vi "Main.vi"() -> ()   [LabVIEW 2017]
uses:
  Acquisition/Hardware Configuration.ctl
  Settings/Settings.ctl
  Logging/Logging Configuration.ctl
  controls/UI Data.ctl
  controls/UI State.ctl
  <userlib>/Circular Buffer/Controls/Circular Buffer Operations.ctl
  <vilib>/Utility/miscctls.llb/LVStringsAndValuesArrayTypeDef.ctl
  <vilib>/measure/maresamp.llb/Resample N Waveforms (continuous).vi
  <userlib>/Circular Buffer/Instance VIs/Circular Buffer(2D Wfm-SGL with Attributes).vi
  <vilib>/Waveform/WDTOps.llb/WDT Number of Waveform Samples DBL.vi
  support/Message Queue/Enqueue Message (Single).vi
  <vilib>/Utility/error.llb/Error Cluster From Error Code.vi
  <vilib>/ErrorRing/Error Ring.xnode
  Acquisition/Acquisition.lvlib
  Logging/Logging.lvlib
  Settings/Settings.lvlib
  support/User Event - Stop/User Event - Stop.lvlib
  support/Message Queue/Message Queue.lvlib
  <userlib>/Circular Buffer/Circular Buffer.lvlib
  <vilib>/measure/NI_MAPro.lvlib
panel:
  out "Hardware Configuration":T1={"DAQmx Channel"="", "Sample Rate"=1000.0, "DAQmx Task"="", "ResetInterp"=FALSE, "GainConstants"=[2.0, 10.0, 1.0, 0.1, 0.01, 0.001], "FilterCoefficients"=[], "ChannelNames"=[], "ActiveChannels"=[], "Display Rate"=1000, "ResponseExtension"=TRUE}
  in  "Settings":bool
  in  "Start":bool
  in  "Trigger":bool caption="Force Trigger"
  out "Scale [mm/s]":u8(slide) max=0 scale=1.0..6.0
  out "Filter [Hz]":u8(slide) caption="Filter" max=0 scale=2.0..4.0
  in  "Autoscale":bool
  out "Status":string
  in  "Range Min":dbl=-10.0 format="%#_3f"
  in  "Range Max":dbl=10.0 format="%#_3f"
  in  "Chart Length[s]":dbl=10.0 min=1.0 max=120.0 step=1.0
  in  "Exit":bool
  out "WD":T2(array[cluster])
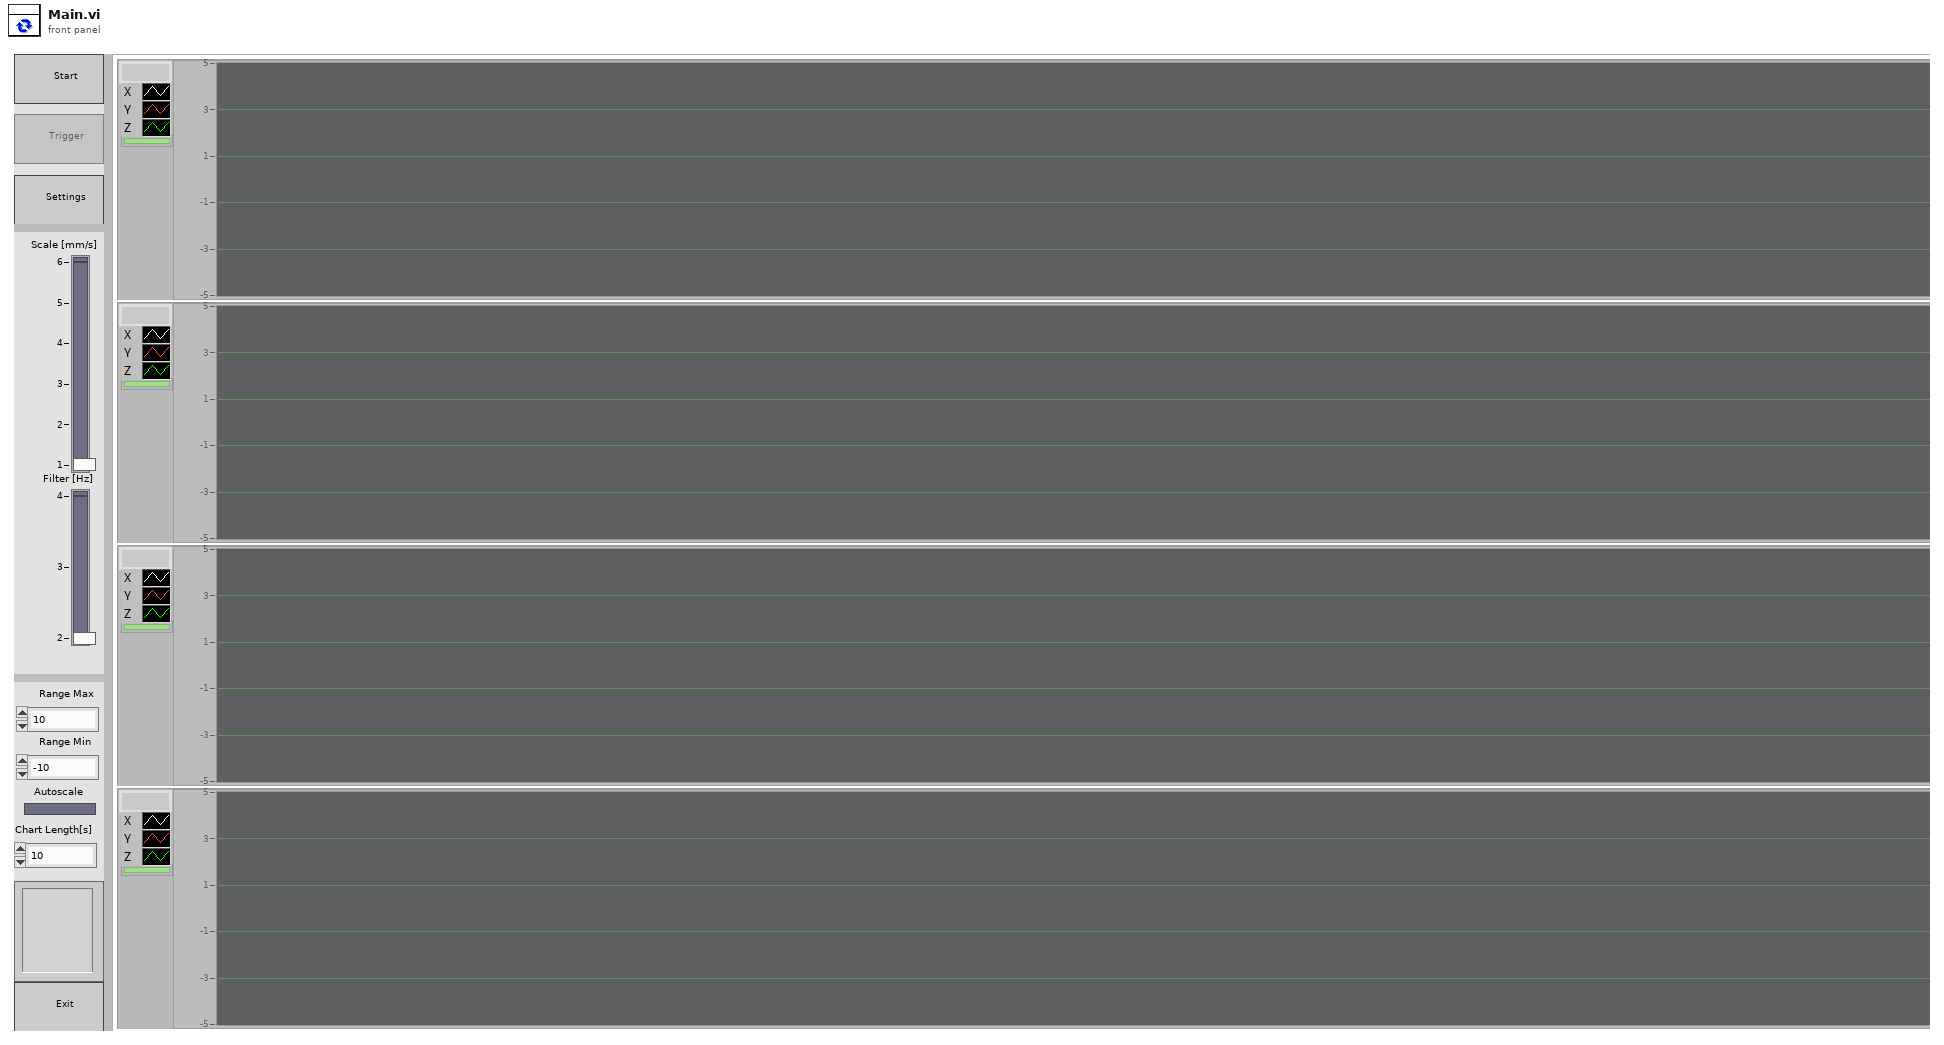
[diagram p1: front panel]
types:
  T1 = typedef "Acquisition.lvlib/Hardware Configuration.ctl" = cluster{"DAQmx Channel":string, "Sample Rate":dbl, "DAQmx Task":refnum<k21>, "ResetInterp":bool, "GainConstants":dbl[], "FilterCoefficients":dbl[][], "ChannelNames":string[], "ActiveChannels":i32[], "Display Rate":i32, "ResponseExtension":bool}
  T2 = cluster{"Graph":waveform(sgl)[], "Name 2":string, "Clip":bool}[]
  T3 = typedef "UI State.ctl" = enum16{"Idle", "Acquiring and Logging", "Waiting for Exit", "Waiting for Exit (Acq Stopped)", "Waiting for Exit (Log Stopped)", "Waiting for Stop", "Waiting for Stop (Acq Stopped)", "Waiting for Stop (Log Stopped)"}
  T4 = typedef "UI Data.ctl" = cluster{"Start Ref":refnum<vi>, "Trigger Ref":refnum<vi>, "Settings Ref":refnum<vi>, "Status Ref":refnum<vi>, "Exit Ref":refnum<vi>, "Data Ref":refnum<vi>}
  T5 = typedef "Settings.lvlib/Settings.ctl" = cluster{"Hardware Configuration":T1, "Logging Configuration":T6}
  T6 = typedef "Logging.lvlib/Logging Configuration.ctl" = cluster{"Log File Base Path":path, "Samples to Save":u32, "Trigger - Threshold":dbl, "Trigger - Channel":u32, "Always Log":bool, "External Trigger":bool, "External Trigger Armed":bool, "TDMS File Reference":refnum<k34>, "DAQVersion":string, "SWVersion":string, "CircSamples":u32, "BeepWhenComplete":bool, "ChannelConfig":string[][], "ActiveChannels":i32[], "Title":string, "Description":string, "ChannelNames":string[], "ResponseExtension":bool}
  T7 = typedef "Message Queue.lvlib/All Message Queues.ctl" = cluster{"UI":refnum<queue>, "Acquisition":refnum<queue>, "Logging":refnum<queue>}
  T8 = typedef "LVRangeTypeDef.ctl" = cluster{"Minimum":dbl, "Maximum":dbl, "Increment":dbl, "Minor Increment":dbl, "Start":dbl}
  T9 = typedef "LVRectTypeDef.ctl" = cluster{"Left":i16, "Top":i16, "Right":i16, "Bottom":i16}
  T10 = typedef "Circular Buffer.lvlib/Circular Buffer Operations.ctl" = enum16{"Initialize", "Get Backlog", "Write", "Read (continuous)", "Read (most recent)", "Peak"}
  T11 = typedef "LVStringsAndValuesArrayTypeDef.ctl" = cluster{"String":string, "Value":ext}[]
  T12 = cluster{"Samples per Channel":u32, "Channels":u32}
  T13 = enum8{"Enabled", "Disabled", "Disabled and Grayed Out"}
  T14 = typedef "LVBoundsTypeDef.ctl" = cluster{"Width":u32, "Height":u32}
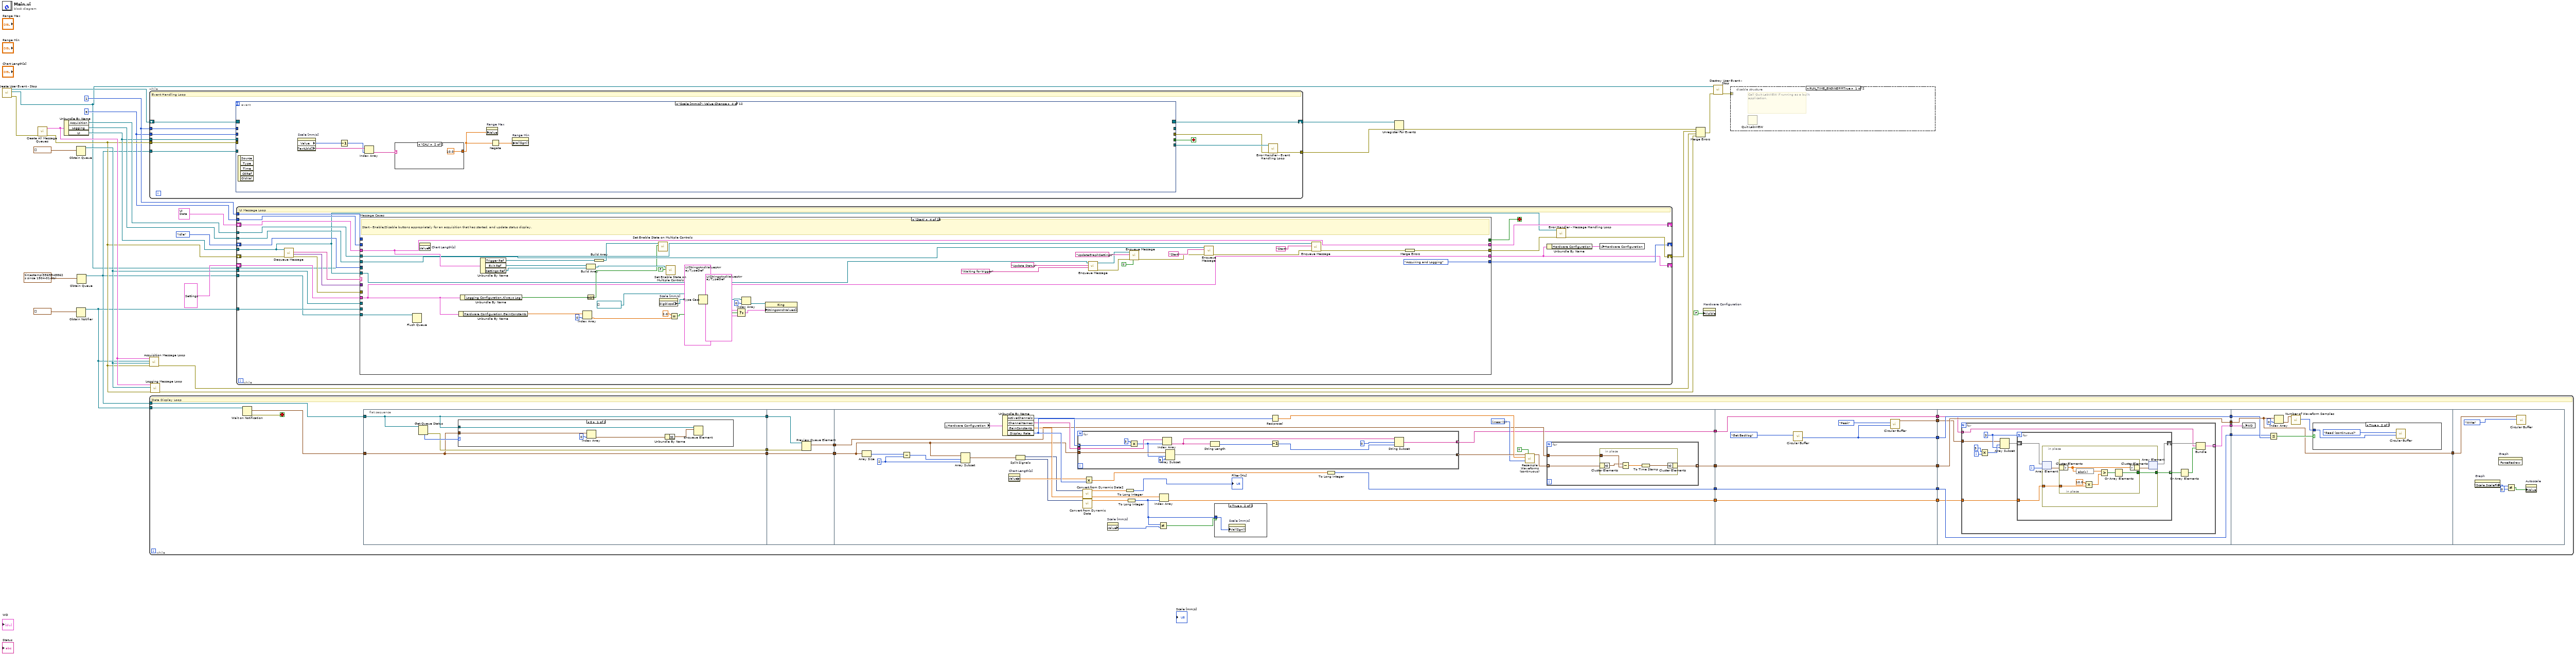
[diagram p0: block diagram]
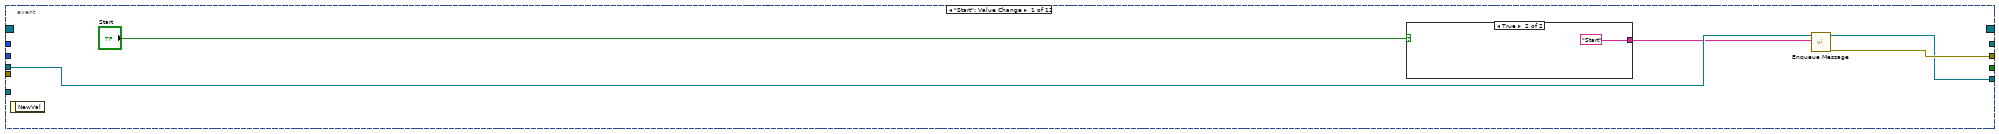
[diagram p6: hidden frame]
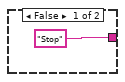
[diagram p7: hidden frame]
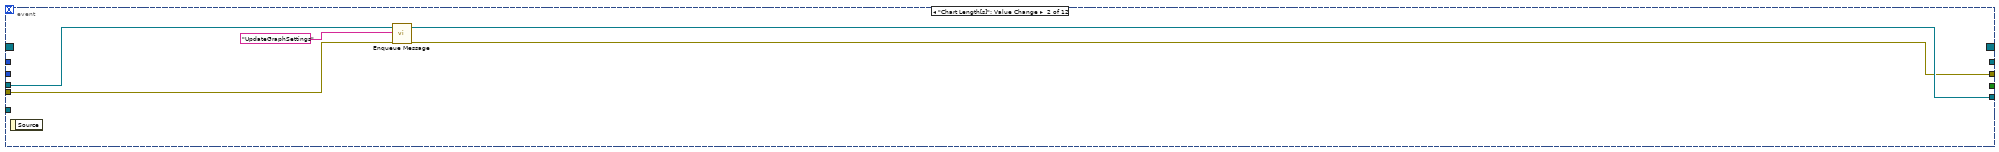
[diagram p8: hidden frame]
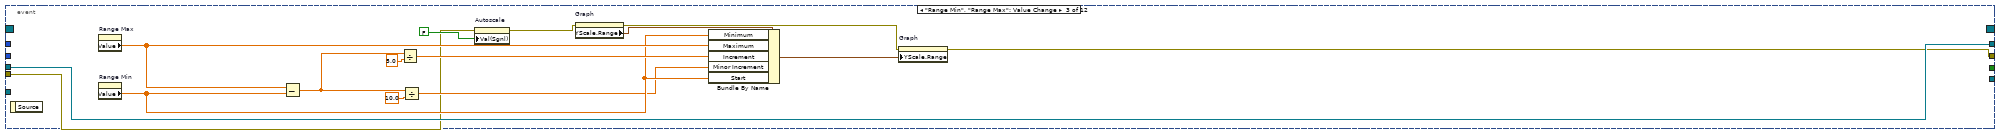
[diagram p9: hidden frame]
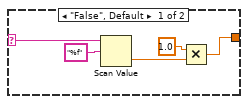
[diagram p10: hidden frame]
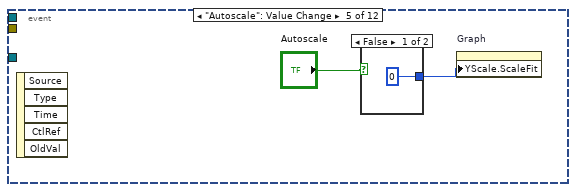
[diagram p11: hidden frame]
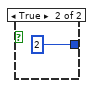
[diagram p12: hidden frame]
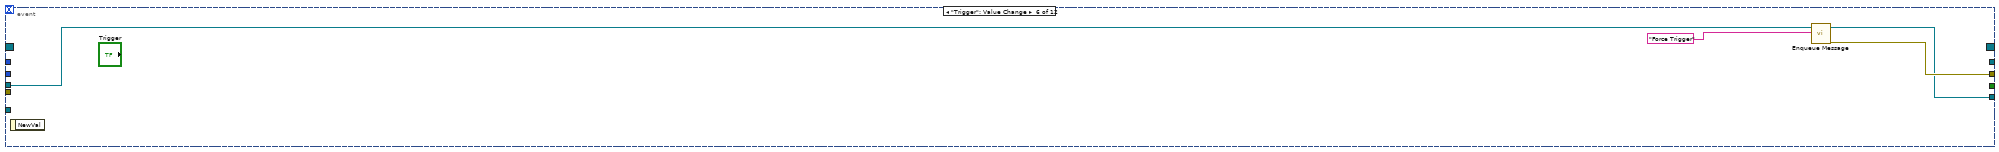
[diagram p13: hidden frame]
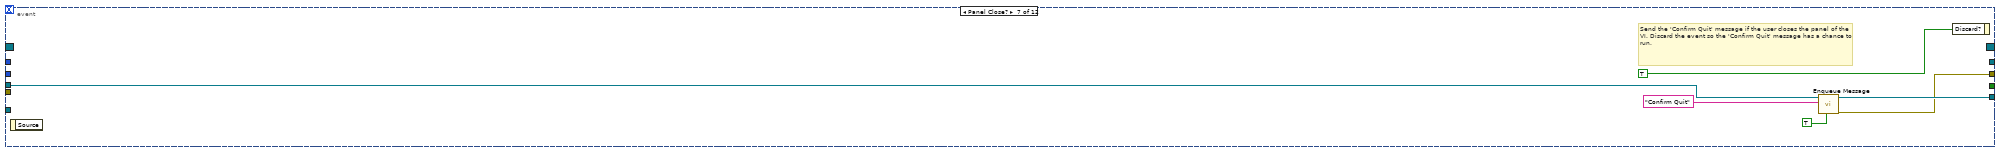
[diagram p14: hidden frame]
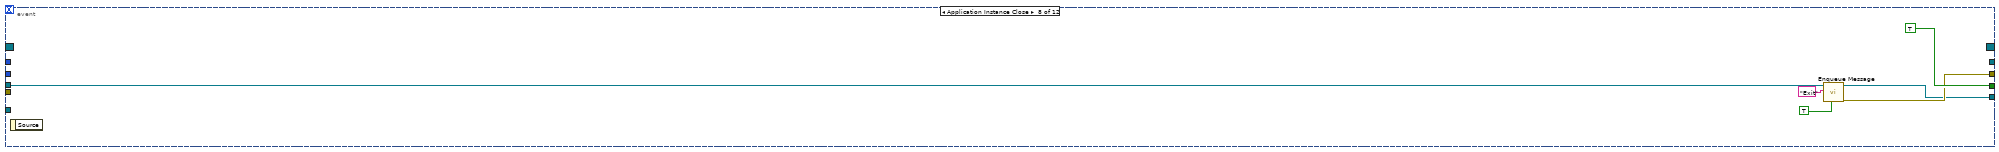
[diagram p15: hidden frame]
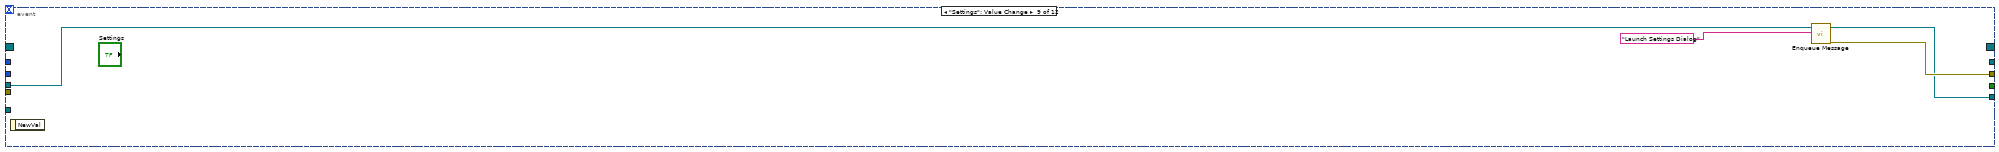
[diagram p16: hidden frame]
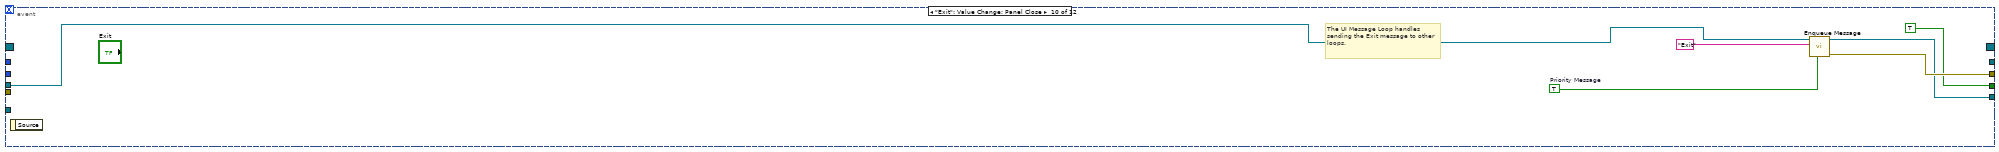
[diagram p17: hidden frame]
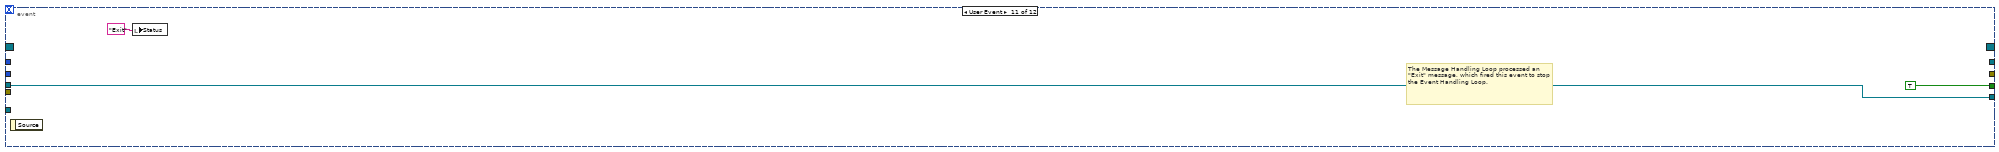
[diagram p18: hidden frame]
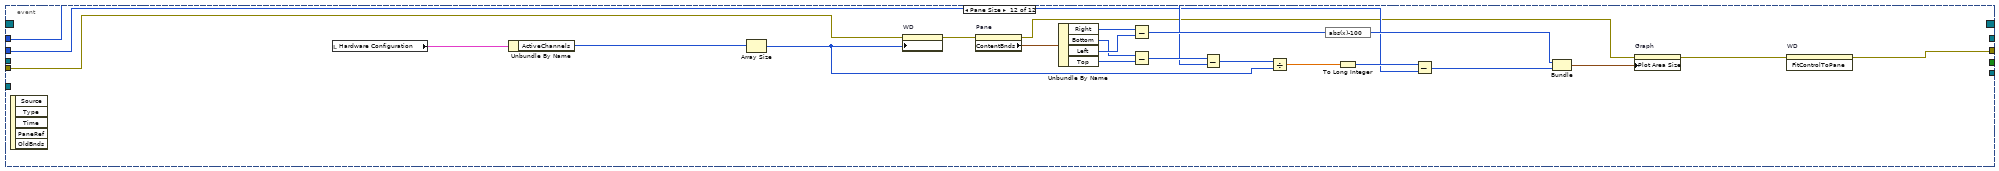
[diagram p19: hidden frame]
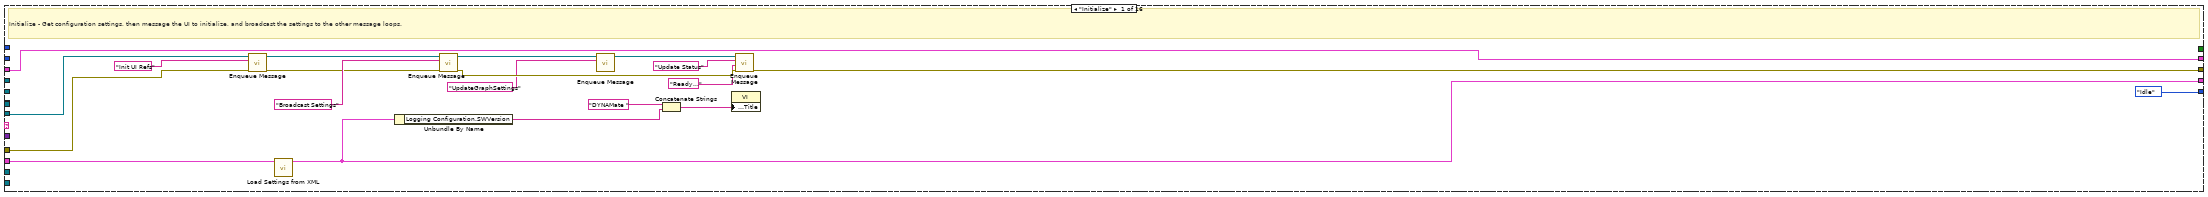
[diagram p20: hidden frame]
diagram:
  w5 = 9 ("y")
  w6 = i16 1 ("y")
  n1 = call "Create User Event - Stop.vi"() -> ("error out"=w23:errorcluster, "User Event - Stop"=w2:refnum<user-event>, "Stop Event Registration Refnum"=w25:refnum<event-registration>)  [unwired: 9 in]
  n2 = call "Create All Message Queues.vi"("error in (no error)"=w23) -> ("error out"=w8:errorcluster, "Message Queues out"=w22:T7)  [unwired: 9 in]
  n3 = Unbundle By Name(w22) -> ("Acquisition"=w17:refnum<queue>, "Logging"=w16:refnum<queue>, "UI"=w10:refnum<queue>)
  n4 = Obtain Queue(element data type=waveform(dbl)[] []) -> (queue out=w13:refnum<queue>)  [unwired: 4 in, 2 out]
  n5 = Obtain Notifier(notification data type=waveform(dbl)[] []) -> (notifier out=w4:refnum<notifier>)  [unwired: 3 in, 2 out]
  n6 = Obtain Queue(element data type=timestamp(3569548862.6211414 s since 1904-01-01) ("seconds since 1Jan1904")) -> (queue out=w3:refnum<queue>)  [unwired: 4 in, 2 out]
  n7 = while {
    tunnel: w10 -> [w38]
    tunnel: [w33] -> w27
    shift-right: [w37] -> w19
    shift-left: w25 -> [w39]
    tunnel: w3 -> [w32]
    tunnel: w8 -> [w31]
    tunnel: w6 -> [w30]
    tunnel: w5 -> [w29]
    stop <- w36 stop-if-true
    # "Event Handling Loop"
    n8 = event shown="[3] \"Scale [mm/s]\": Value Change" {
      selector: w39 -> [_ _ _ _ _ _ _ _ _ _ _ _]
      dyn-events: [_ _ _ _ _ _ _ _ _ _ _ _] -> w37
      timeout: _ -> [_ _ _ _ _ _ _ _ _ _ _ _]
      tunnel: [_ _ _ _ _ _ _ TRUE ("Discard?") _ TRUE ("Discard?") TRUE ("Discard?") _] -> w36
      tunnel: w38 -> [w43 w48 w66 _ _ w85 w92 w96 w100 w105 w109 _]
      tunnel: [w44 w49 w52 _ _ w84 w87 w95 w102 w108 _ w112] -> w34
      tunnel: [w42 w50 _ _ _ w83 w88 w94 w99 w104 w109 _] -> w35
      tunnel: w32 -> [_ _ _ _ _ _ _ _ _ _ _ _]
      tunnel: w31 -> [_ w47 w53 _ _ _ _ _ _ _ _ w122]
      tunnel: w30 -> [_ _ _ _ _ _ _ _ _ _ _ w118]
      tunnel: w29 -> [_ _ _ _ _ _ _ _ _ _ _ w117]
      tunnel: [_ _ w66 _ _ _ _ _ _ _ _ _] -> _
      event "Start": Value Change {
        n9 = event-data() -> ()  [unwired: 1 in, 1 out]
        n10 = case shown="True" "Start" {
          tunnel: ["Stop" ("Message") "Start" ("Message")] -> w40
          frame False {
          }
          frame True {
          }
        }
        n11 = call-poly "Enqueue Message.vi"("Message"=w40, "Message Queue"=w43) -> ("error out"=w44:errorcluster, "dup Message Queue"=w42:refnum<queue>)  [unwired: 8 in]
      }
      event "Chart Length[s]": Value Change {
        n12 = event-data() -> ()  [unwired: 1 in, 1 out]
        n13 = call-poly "Enqueue Message.vi"("error in (no error)"=w47, "Message"="UpdateGraphSettings", "Message Queue"=w48) -> ("error out"=w49:errorcluster, "dup Message Queue"=w50:refnum<queue>)  [unwired: 7 in]
      }
      event "Range Min", "Range Max": Value Change {
        n14 = event-data() -> ()  [unwired: 1 in, 1 out]
        n15 = property on="Range Max" class="DigNum (strict)"() -> ("Value"=w63:dbl)  [unwired: 2 in, 2 out]
        n16 = property on="Range Min" class="DigNum (strict)"() -> ("Value"=w60:dbl)  [unwired: 2 in, 2 out]
        n17 = Subtract(x=w63, y=w60) -> (x-y=w59:dbl)
        n18 = Divide(x=w59, y=5.0) -> (x/y=w61:dbl)
        n19 = Divide(x=w59, y=10.0) -> (x/y=w58:dbl)
        n20 = property on="Autoscale" class="Bool (strict)"(error in=w53, "Val(Sgnl)"=FALSE) -> (error out=w55:errorcluster)  [unwired: 1 in, 1 out]
        n21 = property on="Graph" class="WFGraph (strict)"(error in=w55) -> (error out=w54:errorcluster, "YScale.Range"=w64:T8)  [unwired: 1 in, 1 out]
        n22 = Bundle By Name(cluster=w64, "Minimum"=w60, "Maximum"=w63, "Increment"=w61, "Minor Increment"=w58, "Start"=w60) -> (w65:T8)
        n23 = property on="Graph" class="WFGraph (strict)"(error in=w54, "YScale.Range"=w65) -> (error out=w52:errorcluster)  [unwired: 1 in, 1 out]
      }
      event "Scale [mm/s]": Value Change {
        n24 = event-data() -> ()  [unwired: 1 in, 5 out]
        n25 = property on="Scale [mm/s]" class="Slide (strict)"() -> ("Value"=w71:u8, "TextLbls[]"=w70:string[])  [unwired: 2 in, 2 out]
        n26 = Decrement(x=w71) -> (x-1=w69:u8)
        n27 = Index Array(array=w70, index=w69) -> (element=w68:string)
        n28 = case shown="\"CAL\"" w68 {
          selector: w68 -> [w77 _]
          tunnel: [w74 10.0 ("x")] -> w67
          frame "False", Default {
            n29 = Scan Value(string=w77, format string="%f") -> (value=w75:dbl)  [unwired: 1 in, 1 out]
            n30 = Multiply(x=1.0, y=w75) -> (x*y=w74:dbl)
          }
          frame "CAL" {
          }
        }
        n31 = property on="Range Max" class="DigNum (strict)"("Value"=w67) -> ()  [unwired: 2 in, 2 out]
        n32 = Negate(x=w67) -> (-x=w72:dbl)
        n33 = property on="Range Min" class="DigNum (strict)"("Val(Sgnl)"=w72) -> ()  [unwired: 2 in, 2 out]
      }
      event "Autoscale": Value Change {
        n34 = event-data() -> ()  [unwired: 1 in, 5 out]
        n35 = case shown="False" "Autoscale" {
          tunnel: [0 2] -> w79
          frame False {
          }
          frame True {
          }
        }
        n36 = property on="Graph" class="WFGraph (strict)"("YScale.ScaleFit"=w79) -> ()  [unwired: 2 in, 2 out]
      }
      event "Trigger": Value Change {
        n37 = event-data() -> ()  [unwired: 1 in, 1 out]
        n38 = call-poly "Enqueue Message.vi"("Message"="Force Trigger", "Message Queue"=w85) -> ("error out"=w84:errorcluster, "dup Message Queue"=w83:refnum<queue>)  [unwired: 8 in]
      }
      event Panel Close? {
        # "Send the 'Confirm Quit' message if the user closes the panel of the VI. Discard the event so the 'Confirm Quit' message has a chance to run."
        n39 = event-data() -> ()  [unwired: 1 in, 1 out]
        n40 = call-poly "Enqueue Message.vi"("Priority Message? (F)"=TRUE, "Message"="Confirm Quit", "Message Queue"=w92) -> ("error out"=w87:errorcluster, "dup Message Queue"=w88:refnum<queue>)  [unwired: 7 in]
        n41 = event-data("Discard?"=TRUE) -> ()  [unwired: 1 in, 1 out]
      }
      event Application Instance Close {
        n42 = event-data() -> ()  [unwired: 1 in, 1 out]
        n43 = call-poly "Enqueue Message.vi"("Priority Message? (F)"=TRUE, "Message"="Exit", "Message Queue"=w96) -> ("error out"=w95:errorcluster, "dup Message Queue"=w94:refnum<queue>)  [unwired: 7 in]
      }
      event "Settings": Value Change {
        n44 = event-data() -> ()  [unwired: 1 in, 1 out]
        n45 = call-poly "Enqueue Message.vi"("Message"="Launch Settings Dialog", "Message Queue"=w100) -> ("error out"=w102:errorcluster, "dup Message Queue"=w99:refnum<queue>)  [unwired: 8 in]
      }
      event "Exit": Value Change; Panel Close {
        w106 = TRUE  # Priority Message
        # "The UI Message Loop handles sending the Exit message to other loops."
        n46 = event-data() -> ()  [unwired: 1 in, 1 out]
        n47 = call-poly "Enqueue Message.vi"("Priority Message? (F)"=w106, "Message"="Exit", "Message Queue"=w105) -> ("error out"=w108:errorcluster, "dup Message Queue"=w104:refnum<queue>)  [unwired: 7 in]
      }
      event User Event {
        # "The Message Handling Loop processed an \"Exit\" message, which fired this event to stop the Event Handling Loop."
        n48 = event-data() -> ()  [unwired: 1 in, 1 out]
        n49 = local write "Status"("Exit" ("Exit String")) -> ()
      }
      event Pane Size {
        n50 = event-data() -> ()  [unwired: 1 in, 5 out]
        n51 = local read "Hardware Configuration"() -> (w134:T1)
        n52 = Unbundle By Name(w134) -> ("ActiveChannels"=w133:i32[])
        n53 = Array Size(array=w133) -> (size(s)=w121:i32)
        n54 = property on="WD" class="Arr (strict)"(error in=w122, "Number of Rows"=w121) -> (error out=w115:errorcluster)  [unwired: 1 in, 1 out]
        n55 = property on="Pane" class="Pane"(error in=w115) -> (error out=w116:errorcluster, "ContentBnds"=w114:T9)  [unwired: 1 in, 1 out]
        n56 = Unbundle By Name(w114) -> ("Right"=w128:i16, "Bottom"=w126:i16, "Left"=w129:i16, "Top"=w127:i16)
        n57 = Subtract(x=w128, y=w129) -> (x-y=w130:i16)
        n58 = Subtract(x=w126, y=w127) -> (x-y=w131:i16)
        n59 = Subtract(x=w131, y=w118) -> (x-y=w132:i16)
        n60 = Divide(x=w132, y=w121) -> (x/y=w124:dbl)
        n61 = expression code="abs(x)-100"(w130) -> (w123:i16)
        n62 = To Long Integer(number=w124) -> (32bit integer=w120:i32)
        n63 = Subtract(x=w120, y=w117) -> (x-y=w119:i32)
        n64 = Bundle(w123, w119) -> (w125:cluster{i16, i32})  [unwired: 1 in]
        n65 = property on="Graph" class="WFGraph (strict)"(error in=w116, "Plot Area Size"=w125) -> (error out=w113:errorcluster)  [unwired: 1 in, 1 out]
        n66 = invoke on="WD" class="Arr (strict)" method="FitControlToPane"(error in=w113) -> (error out=w112:errorcluster)  [unwired: 2 in, 2 out]
      }
    }
    n67 = call "Error Handler - Event Handling Loop.vi"("error in (no error)"=w34, "Message Queue"=w35) -> ("dup error in"=w33:errorcluster)  [unwired: 8 in, 1 out]
  }
  n68 = call "Acquisition Message Loop.vi"("error in (no error)"=w8, "Data Queue"=w13, "Data Notifier"=w4, "Message Queues"=w22) -> ("error out"=w24:errorcluster)  [unwired: 7 in]
  n69 = while "Data Display Loop" {
    tunnel: w4 -> [w157]
    tunnel: w3 -> [w153]
    stop <- w158 stop-if-true
    # "Data Display Loop"
    n70 = Wait on Notification(notifier=w157) -> (notification=w154:waveform(dbl)[], error out=w158:errorcluster)  [unwired: 3 in, 2 out]
    n71 = flat-sequence {
      tunnel: w154 -> [w159]
      tunnel: w153 -> [w160]
      tunnel: [w161] -> w152
      tunnel: [w160] -> w150
      tunnel: [w159] -> w149
      tunnel: w152 -> [w171]
      tunnel: [w170] -> w151
      tunnel: w150 -> [w169]
      tunnel: w149 -> [w168]
      tunnel: [w168] -> w148
      tunnel: [w182] -> w155
      tunnel: w151 -> [w180]
      tunnel: w148 -> [w179]
      tunnel: [w178] -> w147
      tunnel: [w177] -> w139
      tunnel: [w176] -> w137
      tunnel: [w226] -> w146
      tunnel: [w228] -> w144
      tunnel: w155 -> [w228]
      tunnel: [w225] -> w142
      tunnel: w147 -> [w225]
      tunnel: [w224] -> w140
      tunnel: w139 -> [w223]
      tunnel: [w223] -> w138
      tunnel: w137 -> [w222]
      tunnel: [w222] -> w136
      tunnel: w146 -> [w236]
      tunnel: [w236] -> w145
      tunnel: w144 -> [w235]
      tunnel: [w235] -> w143
      tunnel: w142 -> [w234]
      tunnel: [w234] -> w141
      tunnel: w140 -> [w233]
      tunnel: w138 -> [w232]
      tunnel: w136 -> [w231]
      tunnel: [w230] -> w135
      tunnel: w145 -> [w268]
      tunnel: w143 -> [w269]
      tunnel: [w269] -> w156
      tunnel: w141 -> [w266]
      tunnel: w135 -> [w265]
      tunnel: w156 -> [w278]
      frame #0 {
        n72 = Get Queue Status(queue=w160) -> (error out=w161:errorcluster, # elements in queue=w162:i32)  [unwired: 2 in, 6 out]
        n73 = case shown="0" w162 {
          tunnel: w160 -> [w163 _]
          tunnel: w159 -> [w164 _]
          frame 0 {
            n74 = Index Array(array=w164, index=0) -> (element=w167:waveform(dbl))
            n75 = Unbundle By Name(w167) -> ("t0"=w166:timestamp)
            n76 = Enqueue Element(queue=w163, element=w166) -> ()  [unwired: 2 in, 3 out]
          }
          frame Default {
          }
        }
      }
      frame #1 {
        n77 = Preview Queue Element(queue=w169, error in (no error)=w171) -> (element=w170:timestamp)  [unwired: 1 in, 3 out]
      }
      frame #2 {
        w184 = u16 1 items=["coerce", "linear", "spline", "FIR filter"] ("interpolation mode")
        w183 = 2 ("length")
        n78 = Array Size(array=w179) -> (size(s)=w193:i32)
        n79 = Subtract(x=w193, y=w183) -> (x-y=w188:i32)
        n80 = local read "Hardware Configuration"() -> (w181:T1)
        n81 = Array Subset(array=w179, index=w188, length=w183) -> (w189:waveform(dbl)[])
        n82 = Unbundle By Name(w181) -> ("ActiveChannels"=w195:i32[], "ChannelNames"=w194:string[], "GainConstants"=w192:dbl[], "Display Rate"=w201:i32)
        n83 = property on="Chart Length[s]" class="DigNum (strict)"() -> ("Value"=w199:dbl)  [unwired: 2 in, 2 out]
        n84 = Split Signals(w189) -> (w190:dynamicdata, w191:dynamicdata)  [unwired: 2 in]
        n85 = for {
          tunnel: w179 -> [w214]
          tunnel: w195 -> [w211] mode=indexing
          tunnel: w194 -> [w210]
          tunnel: [w204] -> w177 mode=indexing
          tunnel: [w203] -> w197 mode=concatenating
          n86 = Multiply(x=3, y=w211) -> (x*y=w209:i32)
          n87 = Index Array(array=w210, index=w209) -> (element=w207:string)
          n88 = Array Subset(array=w214, index=w209, length=3) -> (w203:waveform(dbl)[])
          n89 = String Length(string=w207) -> (length=w206:i32)
          n90 = Decrement(x=w206) -> (x-1=w205:i32)
          n91 = String Subset(string=w207, offset (0)=0, length (rest)=w205) -> (substring=w204:string)
        }
        n92 = call "Convert from Dynamic Data2"("Dynamic Data Type"=w190) -> ("Scalar"=w187:dbl)  [unwired: 3 in]
        n93 = call "Convert from Dynamic Data"("Dynamic Data Type"=w191) -> ("Scalar"=w186:dbl)  [unwired: 3 in]
        n94 = Multiply(x=w199, y=w201) -> (x*y=w196:dbl)
        n95 = property on="Scale [mm/s]" class="Slide (strict)"() -> ("Value"=w173:u8)  [unwired: 2 in, 2 out]
        n96 = To Long Integer(number=w187) -> (32bit integer=→"Filter [Hz]":i32)
        n97 = To Long Integer(number=w186) -> (32bit integer=w174:i32)
        n98 = Not Equal?(x=w174, y=w173) -> (x != y?=w172:bool)
        n99 = Index Array(array=w192, index=w174) -> (element=w176:dbl)
        n100 = case shown="True" w172 {
          tunnel: w174 -> [_ w202]
          frame False {
          }
          frame True {
            n101 = property on="Scale [mm/s]" class="Slide (strict)"("Val(Sgnl)"=w202) -> ()  [unwired: 2 in, 2 out]
          }
        }
        n102 = Reciprocal(x=w201) -> (1/x=w200:dbl)
        n103 = To Long Integer(number=w196) -> (32bit integer=w178:i32)
        n104 = call-poly <vilib>:"Resample Waveforms (continuous).vi"("waveforms in"=w197, "reset"=TRUE, "dt"=w200, "interpolation mode"=w184) -> ("resampled waveforms out"=w198:waveform(dbl)[])  [unwired: 7 in, 4 out]
        n105 = for {
          tunnel: w198 -> [w217] mode=indexing
          tunnel: [w216] -> w182 mode=indexing
          tunnel: w180 -> [w215]
          n106 = in-place {
            in-place-border: w215 -> [w220]
            n107 = in-place-cluster #1(w217) -> ("t0"=w218:timestamp)
            n108 = Subtract(x=w218, y=w220) -> (x-y=w221:dbl)
            n109 = To Time Stamp(1:w221) -> (0:w219:timestamp)
            n110 = in-place-cluster #1("t0"=w219) -> (w216:waveform(dbl))
          }
        }
      }
      frame #3 {
        n111 = call-poly <userlib>:"Circular Buffer.vi"("Operation"=Circular_Buffer_Operations."Get Backlog") -> ("Elements Remaining"=w226:i32)  [unwired: 7 in, 3 out]
        n112 = call-poly <userlib>:"Circular Buffer.vi"("Read Size"=w226, "Operation"=Circular_Buffer_Operations."Peak") -> ("Data Out"=w224:waveform(sgl)[])  [unwired: 6 in, 3 out]
      }
      frame #4 {
        n113 = for {
          tunnel: [w247] -> w230 mode=indexing
          tunnel: w233 -> [w239]
          tunnel: w231 -> [w238]
          tunnel: w232 -> [w237] mode=indexing
          i -> [w243]
          w241 = 3 ("length")
          n114 = Multiply(x=3, y=w243) -> (x*y=w246:i32)
          n115 = Array Subset(array=w239, index=w246, length=w241) -> (w240:waveform(sgl)[])
          n116 = for {
            N: w241 -> [_]
            tunnel: [w253] -> w245 mode=indexing
            shift-right: [w251] -> w242
            shift-left: w240 -> [w250]
            tunnel: w238 -> [w249]
            i -> [w252]
            n117 = in-place {
              in-place-border: [w257] -> w253
              in-place-border: w249 -> [w254]
              n118 = in-place-array #2(w250, w252) -> (w256:waveform(sgl))
              n119 = in-place {
                in-place-border: w254 -> [w264]
                in-place-border: [w259] -> w257
                n120 = in-place-cluster #3(w256) -> ("Y"=w260:sgl[])
                n121 = expression code="abs(x)"(w260) -> (w258:sgl[])
                n122 = Multiply(x=10.0, y=w264) -> (x*y=w262:dbl)
                n123 = Greater?(x=w258, y=w262) -> (0:w263:bool[])
                n124 = Or Array Elements(Boolean array=w263) -> (logical OR=w259:bool)
                n125 = in-place-cluster #3("Y"=w260) -> (w255:waveform(sgl))
              }
              n126 = in-place-array #2(w255) -> (w251:waveform(sgl)[])  [unwired: 1 out]
            }
          }
          n127 = Or Array Elements(Boolean array=w245) -> (logical OR=w244:bool)
          n128 = Bundle(w242, "String"=w237, w244) -> (w247:cluster{waveform(sgl)[], "String":string, bool})  [unwired: 1 in]
        }
      }
      frame #5 {
        n129 = local write "WD"(w265) -> ()
        n130 = Less Or Equal?(x=w266, y=w268) -> (x <= y?=w271:bool)
        n131 = Index Array(array=w269, index=0) -> (element=w272:waveform(dbl))
        n132 = call-poly <vilib>:"Number of Waveform Samples.vi"("waveform in"=w272) -> ("number of samples"=w267:i32)  [unwired: 8 in, 2 out]
        n133 = case shown="True" w271 {
          tunnel: w267 -> [_ w273]
          frame False {
          }
          frame True {
            n134 = call-poly <userlib>:"Circular Buffer.vi"("Read Size"=w273, "Operation"=Circular_Buffer_Operations."Read (continuous)") -> ()  [unwired: 6 in, 4 out]
          }
        }
      }
      frame #6 {
        n135 = property on="Graph" class="WFGraph (strict)"() -> ("YScale.ScaleFit"=w277:u8)  [unwired: 2 in, 2 out]
        n136 = invoke on="Graph" class="WFGraph (strict)" method="ForceRedraw"() -> ()  [unwired: 3 in, 3 out]
        n137 = Not Equal?(x=w277, y=u8 0) -> (x != y?=w275:bool)
        n138 = call-poly <userlib>:"Circular Buffer.vi"("Operation"=Circular_Buffer_Operations."Write", "Data In"=w278) -> ()  [unwired: 6 in, 4 out]
        n139 = property on="Autoscale" class="Bool (strict)"("Value"=w275) -> ()  [unwired: 2 in, 2 out]
      }
    }
  }
  n140 = call "Logging Message Loop.vi"("error in (no error)"=w8, "Data Queue"=w13, "Message Queues"=w22) -> ("error out"=w21:errorcluster)  [unwired: 8 in]
  n141 = while {
    tunnel: w10 -> [w281]
    shift-right: [w289] -> w28
    shift-left: w8 -> [w301]
    shift-right: [w283] -> _
    shift-left: T5 {"Hardware Configuration"={"DAQmx Channel"="", "Sample Rate"=1000.0, "DAQmx Task"="", "ResetInterp"=FALSE, "GainConstants"=[2.0, 10.0, 1.0, 0.1, 0.01, 0.001], "FilterCoefficients"=[], "ChannelNames"=["CH1X", "CH1Y", "CH1Z", "CH2X", "CH2Y", "CH2Z", "CH3X", "CH3Y", "CH3Z", "CH4X", "CH4Y", "CH4Z", "CH5X", "CH5Y", "CH5Z", "CH6X", "CH6Y", "CH6Z", "CH7X", "CH7Y", "CH7Z", "CH8X", "CH8Y", "CH8Z"], "ActiveChannels"=[0, 1, 2, 3, 4, 5, 6, 7], "Display Rate"=250, "ResponseExtension"=FALSE}, "Logging Configuration"={"Log File Base Path"=path "c:/data.tdms", "Samples to Save"=9900, "Trigger - Threshold"=0.0, "Trigger - Channel"=0, "Always Log"=FALSE, "External Trigger"=TRUE, "External Trigger Armed"=FALSE, "TDMS File Reference"=refnum, "DAQVersion"="", "SWVersion"="", "CircSamples"=100, "BeepWhenComplete"=FALSE, "ChannelConfig"=[["CH1", "CH1", "NA", "XYZ"], ["CH2", "CH2", "NA", "XYZ"], ["CH3", "CH3", "NA", "XYZ"], ["CH4", "CH4", "NA", "XYZ"], ["CH5", "CH5", "NA", "XYZ"], ["CH6", "CH6", "NA", "XYZ"], ["CH7", "CH7", "NA", "XYZ"], ["CH8", "CH8", "NA", "XYZ"]], "ActiveChannels"=[0, 1, 2, 3, 4, 5, 6, 7], "Title"="", "Description"="", "ChannelNames"=["CH1X", "CH1Y", "CH1Z", "CH2X", "CH2Y", "CH2Z", "CH3X", "CH3Y", "CH3Z", "CH4X", "CH4Y", "CH4Z", "CH5X", "CH5Y", "CH5Z", "CH6X", "CH6Y", "CH6Z", "CH7X", "CH7Y", "CH7Z", "CH8X", "CH8Y", "CH8Z"], "ResponseExtension"=TRUE}} ("Settings") -> [w297]
    shift-right: [w295] -> _
    shift-left: T4 {"Start Ref"=refnum, "Trigger Ref"=refnum, "Settings Ref"=refnum, "Status Ref"=refnum, "Exit Ref"=refnum, "Data Ref"=refnum} ("Measurement UI Controls") -> [w296]
    tunnel: w17 -> [w294]
    tunnel: w16 -> [w293]
    tunnel: w4 -> [w292]
    tunnel: w13 -> [w291]
    shift-right: [w287] -> _
    shift-left: UI_State."Idle" ("UI State") -> [w288]
    tunnel: w3 -> [w286]
    tunnel: w6 -> [w285]
    tunnel: w5 -> [w284]
    tunnel: w2 -> [w280]
    stop <- w302 stop-if-true
    # "UI Message Loop"
    n142 = call "Dequeue Message.vi"("error in (no error)"=w301, "Message Queue"=w281) -> ("error out"=w300:errorcluster, "Message Data"=w298:variant, "Message"=w299:string)  [unwired: 6 in, 1 out]
    n143 = case "Message Cases" shown="\"Start\"" w299 {
      selector: w299 -> [_ _ _ _ _ _ _ _ _ _ _ _ _ _ _ w645]
      tunnel: w281 -> [w315 _ _ w399 _ w409 w436 w461 _ w504 w522 w532 w567 _ _ _]
      tunnel: w300 -> [w314 w338 w349 _ w405 w430 w438 w463 w486 w506 w526 w531 w573 w579 w623 _]
      tunnel: [w321 w338 w350 w400 w408 w431 w437 w462 w498 w499 w517 w530 w558 w578 w595 w646] -> w290
      tunnel: [_ _ _ _ _ _ _ _ _ _ _ _ TRUE _ _ _] -> w302
      tunnel: w298 -> [_ _ w348 _ _ _ _ _ _ _ w525 _ _ _ _ _]
      tunnel: [w306 w337 w340 w379 w407 w429 w442 w467 w496 w500 w528 w535 w572 w577 w580 w648] -> w283
      tunnel: w297 -> [w307 w337 w340 w379 w407 w429 w442 w467 w496 w507 w528 w535 w572 w577 w580 w648]
      tunnel: w296 -> [w317 w336 w346 w396 w406 w426 w441 w466 w492 w502 w527 w534 w570 w576 w622 w647]
      tunnel: [w317 w335 w346 w396 w406 w426 w441 w466 w492 w502 w527 w534 w570 w576 w622 w647] -> w295
      tunnel: w294 -> [_ _ _ w386 _ w415 _ _ w491 _ _ _ w569 _ _ _]
      tunnel: w293 -> [_ _ _ w389 w402 w418 _ _ w490 _ _ _ w568 _ _ _]
      tunnel: w292 -> [_ _ _ _ _ _ _ _ _ _ _ _ w566 _ _ _]
      tunnel: w291 -> [_ _ _ _ _ _ _ _ _ _ _ _ w563 _ _ _]
      tunnel: w288 -> [_ _ w342 _ w401 w413 w440 w465 w489 w501 w516 w533 _ w575 w621 w644]
      tunnel: [UI_State."Idle" ("UI State") UI_State."Idle" ("UI State") w342 UI_State."Acquiring and Logging" ("UI State") w401 w412 w439 w464 w489 w501 w516 w529 UI_State."Idle" ("UI State") w575 w621 w644] -> w287
      tunnel: w286 -> [_ _ _ w382 _ _ _ _ _ _ _ _ _ _ _ _]
      tunnel: w285 -> [_ _ _ _ _ _ _ _ _ _ _ _ _ _ w600 _]
      tunnel: w284 -> [_ _ _ _ _ _ _ _ _ _ _ _ _ _ w599 _]
      tunnel: w280 -> [_ _ _ _ _ _ _ _ _ _ _ _ w557 _ _ _]
      frame "Initialize" {
        # "Initialize - Get configuration settings, then message the UI to initialize, and broadcast the settings to the other message loops."
        n144 = call-poly "Enqueue Message.vi"("error in (no error)"=w314, "Message"="Init UI Refs", "Message Queue"=w315) -> ("error out"=w312:errorcluster, "dup Message Queue"=w313:refnum<queue>)  [unwired: 7 in]
        n145 = call "Load Settings from XML.vi"("Settings in"=w307) -> ("Settings out"=w306:T5)  [unwired: 9 in, 1 out]
        n146 = Unbundle By Name(w306) -> ("Logging Configuration.SWVersion"=w310:string)
        n147 = call-poly "Enqueue Message.vi"("error in (no error)"=w312, "Message"="Broadcast Settings", "Message Queue"=w313) -> ("error out"=w322:errorcluster, "dup Message Queue"=w304:refnum<queue>)  [unwired: 7 in]
        n148 = call-poly "Enqueue Message.vi"("Message"="UpdateGraphSettings", "Message Queue"=w304) -> ("dup Message Queue"=w303:refnum<queue>)  [unwired: 8 in, 1 out]
        n149 = Concatenate Strings("DYNAMate " ("string"), w310) -> (w308:string)
        n150 = property on="Property Node" class="VI"("Front Panel.Title"=w308) -> ()  [unwired: 2 in, 2 out]
        n151 = call-poly "Enqueue Message.vi"("error in (no error)"=w322, "Message Data"="Ready..." ("Ready..."), "Message"="Update Status", "Message Queue"=w303) -> ("error out"=w321:errorcluster)  [unwired: 6 in, 1 out]
      }
      frame "Init UI Refs" {
        # "Init UI Refs - Store control references for UI controls.  Also enable/disable controls appropriately."
        n152 = control-ref of="Start"() -> (w327:refnum<vi>)
        n153 = control-ref of="Trigger"() -> (w323:refnum<vi>)
        n154 = control-ref of="Settings"() -> (w330:refnum<vi>)
        n155 = control-ref of="Exit"() -> (w329:refnum<vi>)
        n156 = control-ref of="Status"() -> (w333:refnum<vi>)
        n157 = property class="VI"("Front Panel.Closeable"=TRUE ("Front Panel Window:Closeable")) -> ()  [unwired: 2 in, 2 out]
        n158 = property class="Bool (strict)"(reference=w327, "Value"=FALSE) -> ()  [unwired: 1 in, 2 out]
        n159 = Bundle By Name(cluster=w336, "Start Ref"=w327, "Trigger Ref"=w323, "Settings Ref"=w330, "Status Ref"=w333, "Exit Ref"=w329) -> (w335:T4)
        n160 = Build Array(w329, w330) -> (w332:refnum<vi>[])
        n161 = Build Array(w323) -> (w324:refnum<vi>[])
        n162 = call "Set Enable State on Multiple Controls.vi"("Enable?"=FALSE ("Value"), "Controls"=w324) -> ()  [unwired: 10 in]
        n163 = call "Set Enable State on Multiple Controls.vi"("Enable?"=TRUE, "Controls"=w332) -> ()  [unwired: 10 in]
      }
      frame "Update Status" {
        # "Update Display - Convert the message data to a string to display in the Status indicator."
        n164 = Unbundle By Name(w346) -> ("Trigger Ref"=w343:refnum<vi>, "Settings Ref"=w345:refnum<vi>)
        n165 = Variant To Data(error in=w349, type="", Variant=w348) -> (data=w339:string, error out=w341:errorcluster)
        n166 = local write "Status"(w339) -> ()
        n167 = property class="Bool"(reference=w345) -> ("DisabledEnum"=w344:T13)  [unwired: 1 in, 2 out]
        n168 = case shown="\"Disabled\", Default" w344 {
          tunnel: w339 -> [_ w353 w356]
          tunnel: w343 -> [_ w354 w357]
          frame "Enabled" {
          }
          frame "Disabled and Grayed Out" {
            # "Disable the Force Trigger only while we are logging."
            n169 = Build Array(w354) -> (w355:refnum<vi>[])
            n170 = Not Equal?(x="Logging" ("Logging"), y=w353) -> (x != y?=w351:bool)
            n171 = call "Set Enable State on Multiple Controls.vi"("Enable?"=w351, "Controls"=w355) -> ()  [unwired: 10 in]
          }
          frame "Disabled", Default {
            n172 = Build Array(w357) -> (w359:refnum<vi>[])
            n173 = Not Equal?(x="Logging" ("Logging"), y=w356) -> (x != y?=w360:bool)
            n174 = call "Set Enable State on Multiple Controls.vi"("Enable?"=w360, "Controls"=w359) -> ()  [unwired: 10 in]
          }
        }
        n175 = Merge Errors(w341) -> (w350:errorcluster)
      }
      frame "Start" {
        # "Start - Enable/Disable buttons appropriately for an acquisition that has started, and update status display."
        n176 = Flush Queue(queue=w382) -> ()  [unwired: 1 in, 3 out]
        n177 = property on="Chart Length[s]" class="DigNum (strict)" props=["Value"]() -> ()  [unwired: 2 in, 3 out]
        n178 = Unbundle By Name(w379) -> ("Hardware Configuration.GainConstants"=w377:dbl[])
        n179 = Unbundle By Name(w379) -> ("Logging Configuration.Always Log"=w381:bool)
        n180 = Unbundle By Name(w396) -> ("Trigger Ref"=w384:refnum<vi>, "Exit Ref"=w392:refnum<vi>, "Settings Ref"=w391:refnum<vi>)
        n181 = Index Array(array=w377, index=0) -> (element=w376:dbl)
        n182 = Not(x=w381) -> (.not. x?=w380:bool)
        n183 = Build Array(w392, w391) -> (w394:refnum<vi>[])
        n184 = Build Array(w384) -> (w393:refnum<vi>[])
        n185 = call "Set Enable State on Multiple Controls.vi"("Enable?"=w380, "Controls"=w393) -> ()  [unwired: 10 in]
        n186 = property on="Scale [mm/s]" class="Slide (strict)"() -> ("DigDisps[]"=w373:refnum<vi>[])  [unwired: 2 in, 2 out]
        n187 = call "Set Enable State on Multiple Controls.vi"("Enable?"=FALSE, "Controls"=w394) -> ()  [unwired: 10 in]
        n188 = Equal?(x=2.0, y=w376) -> (x = y?=w374:bool)
        n189 = Type Cast(type=refnum<vi>[] [], x=w373) -> (*(type *) &x=w370:refnum<vi>[])
        n190 = Select(t=T11 [{"String"="CAL", "Value"=1.0}, {"String"="100", "Value"=2.0}, {"String"="10", "Value"=3.0}, {"String"="1", "Value"=4.0}, {"String"="0.1", "Value"=5.0}, {"String"="0.01", "Value"=6.0}] ("Strings And Values []"), s=w374, f=T11 [{"String"="CAL", "Value"=1.0}, {"String"="100", "Value"=2.0}, {"String"="10", "Value"=3.0}, {"String"="1", "Value"=4.0}, {"String"="0.1", "Value"=0.0}] ("Strings And Values []")) -> (s? t:f=w368:T11)
        n191 = Index Array(array=w370, index=0) -> (element=w369:refnum<vi>)
        n192 = property class="Ring"(reference=w369, "StringsAndValues[]"=w368) -> ()  [unwired: 1 in, 2 out]
        n193 = call-poly "Enqueue Message.vi"("Message Data"="Waiting for trigger" ("Waiting for trigger"), "Message"="Update Status", "Message Queue"=w399) -> ("error out"=w362:errorcluster, "dup Message Queue"=w363:refnum<queue>)  [unwired: 7 in]
        n194 = call-poly "Enqueue Message.vi"("Priority Message? (F)"=TRUE, "error in (no error)"=w362, "Message"="UpdateGraphSettings", "Message Queue"=w363) -> ("error out"=w361:errorcluster)  [unwired: 6 in, 1 out]
        n195 = call-poly "Enqueue Message.vi"("error in (no error)"=w361, "Message"="Start", "Message Queue"=w389) -> ("error out"=w388:errorcluster)  [unwired: 7 in, 1 out]
        n196 = call-poly "Enqueue Message.vi"("error in (no error)"=w388, "Message"="Start", "Message Queue"=w386) -> ("error out"=w387:errorcluster)  [unwired: 7 in, 1 out]
        n197 = Merge Errors(w387) -> (w400:errorcluster)
      }
      frame "Force Trigger" {
        # "Force Trigger - send a message to the Logging message loop to start logging."
        n198 = call-poly "Enqueue Message.vi"("error in (no error)"=w405, "Message"="Force Trigger", "Message Queue"=w402) -> ("error out"=w404:errorcluster)  [unwired: 7 in, 1 out]
        n199 = Merge Errors(w404) -> (w408:errorcluster)
      }
      frame "Stop" {
        # "Stop - Enable/Disable buttons appropriately for an acquisition that has stopped, and update status display."
        n200 = case shown="\"Waiting for Exit\"" w413 {
          selector: w413 -> [_ w435]
          tunnel: [UI_State."Waiting for Stop" ("UI State") w435] -> w412
          tunnel: w409 -> [_ w433]
          frame Default {
          }
          frame "Waiting for Exit" {
            n201 = call-poly "Enqueue Message.vi"("Message"="Exit", "Message Queue"=w433) -> ()  [unwired: 8 in, 2 out]
          }
        }
        n202 = call-poly "Enqueue Message.vi"("error in (no error)"=w430, "Message Data"="Ready..." ("Ready..."), "Message"="Update Status", "Message Queue"=w409) -> ("error out"=w420:errorcluster)  [unwired: 6 in, 1 out]
        n203 = Unbundle By Name(w426) -> ("Trigger Ref"=w411:refnum<vi>, "Exit Ref"=w422:refnum<vi>, "Settings Ref"=w421:refnum<vi>)
        n204 = Build Array(w422, w421) -> (w424:refnum<vi>[])
        n205 = Build Array(w411) -> (w410:refnum<vi>[])
        n206 = call-poly "Enqueue Message.vi"("error in (no error)"=w420, "Message"="Stop", "Message Queue"=w418) -> ("error out"=w417:errorcluster)  [unwired: 7 in, 1 out]
        n207 = call "Set Enable State on Multiple Controls.vi"("Enable?"=FALSE, "Controls"=w410) -> ()  [unwired: 10 in]
        n208 = call "Set Enable State on Multiple Controls.vi"("Enable?"=TRUE, "Controls"=w424) -> ()  [unwired: 10 in]
        n209 = call-poly "Enqueue Message.vi"("error in (no error)"=w417, "Message"="Stop", "Message Queue"=w415) -> ("error out"=w416:errorcluster)  [unwired: 7 in, 1 out]
        n210 = Merge Errors(w416) -> (w431:errorcluster)
      }
      frame "Acquisition Stopped" {
        # "Logic for determining what action to take when the acquisition has stopped."
        n211 = case shown="\"Waiting for Exit (Log Stopped)\"" w440 {
          selector: w440 -> [w444 _ _ _ _]
          tunnel: [w444 UI_State."Waiting for Exit (Acq Stopped)" ("UI State") UI_State."Waiting for Stop (Acq Stopped)" ("UI State") UI_State."Idle" ("UI State") UI_State."Idle" ("UI State")] -> w439
          tunnel: w438 -> [w443 w445 w447 w453 w459]
          tunnel: [w443 w445 w447 w452 w458] -> w437
          tunnel: w436 -> [_ _ _ w451 w457]
          frame Default {
          }
          frame "Waiting for Exit", "Waiting for Exit (Acq Stopped)" {
          }
          frame "Waiting for Stop", "Waiting for Stop (Acq Stopped)" {
          }
          frame "Waiting for Exit (Log Stopped)" {
            # "If we are waiting to exit, and the logging has already stopped, then the \"Acquisition Stopped\" message indicates that it is time to exit."
            n212 = call-poly "Enqueue Message.vi"("Priority Message? (F)"=TRUE, "error in (no error)"=w453, "Message"="Exit", "Message Queue"=w451) -> ("error out"=w452:errorcluster)  [unwired: 6 in, 1 out]
          }
          frame "Waiting for Stop (Log Stopped)" {
            n213 = call-poly "Enqueue Message.vi"("error in (no error)"=w459, "Message Data"="Ready..." ("Message"), "Message"="Update Status", "Message Queue"=w457) -> ("error out"=w458:errorcluster)  [unwired: 6 in, 1 out]
          }
        }
      }
      frame "Logging Stopped" {
        # "Logic for determining what action to take when the logging has stopped."
        n214 = case shown="\"Waiting for Exit (Acq Stopped)\"" w465 {
          selector: w465 -> [w469 _ _ _ _]
          tunnel: [w469 UI_State."Waiting for Exit (Log Stopped)" ("UI State") UI_State."Waiting for Stop (Log Stopped)" ("UI State") UI_State."Idle" ("UI State") UI_State."Idle" ("UI State")] -> w464
          tunnel: w463 -> [w468 w470 w472 w478 w484]
          tunnel: [w468 w470 w472 w477 w483] -> w462
          tunnel: w461 -> [_ _ _ w476 w482]
          frame Default {
          }
          frame "Waiting for Exit", "Waiting for Exit (Log Stopped)" {
          }
          frame "Waiting for Stop", "Waiting for Stop (Log Stopped)" {
          }
          frame "Waiting for Exit (Acq Stopped)" {
            # "If we are waiting to exit, and the acquisition has already stopped, then the \"Logging Stopped\" message indicates that it is time to exit."
            n215 = call-poly "Enqueue Message.vi"("Priority Message? (F)"=TRUE, "error in (no error)"=w478, "Message"="Exit", "Message Queue"=w476) -> ("error out"=w477:errorcluster)  [unwired: 6 in, 1 out]
          }
          frame "Waiting for Stop (Acq Stopped)" {
            n216 = call-poly "Enqueue Message.vi"("error in (no error)"=w484, "Message Data"="Ready..." ("Message"), "Message"="Update Status", "Message Queue"=w482) -> ("error out"=w483:errorcluster)  [unwired: 6 in, 1 out]
          }
        }
      }
      frame "Broadcast settings" {
        w493 = "Update Settings" ("Message")
        # "Send the 'Update Settings' message to the Logging and Acquisition message loops."
        n217 = Unbundle By Name(w496) -> ("Hardware Configuration"=w488:T1, "Logging Configuration"=w495:T6)
        n218 = call-poly "Enqueue Message.vi"("Message Data"=w488, "Message"=w493, "Message Queue"=w491) -> ("error out"=w497:errorcluster)  [unwired: 7 in, 1 out]
        n219 = invoke on="WD" class="Arr (strict)" method="FitControlToPane"() -> (error out=w487:errorcluster)  [unwired: 3 in, 2 out]
        n220 = call-poly "Enqueue Message.vi"("error in (no error)"=w497, "Message Data"=w495, "Message"=w493, "Message Queue"=w490) -> ("error out"=w494:errorcluster)  [unwired: 6 in, 1 out]
        n221 = Merge Errors(w487, w494, w486) -> (w498:errorcluster)
      }
      frame "Launch Settings Dialog" {
        # "Launch the Settings Dialog when the user clicks the 'Settings' button."
        n222 = call "Settings Dialog.vi"("error in (no error)"=w506, "Settings in"=w507) -> ("error out"=w503:errorcluster, "Cancelled?"=w505:bool, "Settings out"=w500:T5)  [unwired: 6 in, 1 out]
        n223 = case shown="False" w505 {
          tunnel: w504 -> [w511 _]
          tunnel: w503 -> [w514 w515]
          tunnel: [w512 w515] -> w499
          frame False {
            n224 = call-poly "Enqueue Message.vi"("Message"="UpdateGraphSettings", "Message Queue"=w511) -> ("dup Message Queue"=w510:refnum<queue>)  [unwired: 8 in, 1 out]
            n225 = call-poly "Enqueue Message.vi"("Priority Message? (F)"=TRUE, "error in (no error)"=w514, "Message"="Broadcast Settings", "Message Queue"=w510) -> ("error out"=w512:errorcluster)  [unwired: 6 in, 1 out]
          }
          frame True {
          }
        }
      }
      frame "Error" {
        # "Error - Check the error message data and respond accordingly. This message is sent by the \"Error Handler\" VIs at the end of each loop in this application."
        n226 = Variant To Data(error in=w526, type=errorcluster {"status"=FALSE, "code"=0, "source"=""} ("error out"), Variant=w525) -> (data=w523:errorcluster, error out=w519:errorcluster)
        n227 = call <vilib>:"Simple Error Handler.vi"("error in (no error)"=w523) -> ()  [unwired: 4 in, 5 out]
        n228 = call-poly "Enqueue Message.vi"("Priority Message? (F)"=TRUE, "Message"="Exit", "Message Queue"=w522) -> ("error out"=w518:errorcluster)  [unwired: 7 in, 1 out]
        n229 = Merge Errors(w518, w519) -> (w517:errorcluster)
      }
      frame "Confirm Quit" {
        # "Confirm Quit - Message that can confirm whether or not the user wants to exit the application."
        n230 = case shown="\"Acquiring and Logging\"" w533 {
          tunnel: w532 -> [w540 w546]
          tunnel: w531 -> [w539 w544]
          tunnel: [w536 w543] -> w530
          tunnel: [UI_State."Idle" ("UI State") w542] -> w529
          frame Default {
            # "If 'Confirm Quit' comes in while the system is idle, there is no need for a confirmation message."
            n231 = call-poly "Enqueue Message.vi"("Priority Message? (F)"=TRUE, "error in (no error)"=w539, "Message"="Exit", "Message Queue"=w540) -> ("error out"=w536:errorcluster)  [unwired: 6 in, 1 out]
          }
          frame "Acquiring and Logging" {
            n232 = Two Button Dialog(message="Are you sure you want to quit while the acquisition is running?" ("Confirm Quit Message"), 1:"No" ("No"), 2:"Yes" ("Yes")) -> (T button?=w545:bool)
            n233 = case shown="True" w545 {
              tunnel: w546 -> [_ w556]
              tunnel: w544 -> [w550 w555]
              tunnel: [w550 w554] -> w543
              tunnel: [UI_State."Acquiring and Logging" ("UI State") UI_State."Waiting for Exit" ("UI State")] -> w542
              frame False {
                # "User did not want to quit."
              }
              frame True {
                n234 = call-poly "Enqueue Message.vi"("error in (no error)"=w555, "Message"="Stop", "Message Queue"=w556) -> ("error out"=w554:errorcluster)  [unwired: 7 in, 1 out]
              }
            }
          }
        }
      }
      frame "Exit" {
        w571 = "Exit" ("Message")
        # "Stop the VI"
        # "Exit - Fire the User Event to stop the Event Handling Loop.  Also send Exit messages to the Acquisition and Logging loops."
        n235 = call-poly "Enqueue Message.vi"("Priority Message? (F)"=TRUE, "Message"=w571, "Message Queue"=w569) -> ()  [unwired: 7 in, 2 out]
        n236 = call-poly "Enqueue Message.vi"("Priority Message? (F)"=TRUE, "Message"=w571, "Message Queue"=w568) -> ()  [unwired: 7 in, 2 out]
        n237 = Release Queue(queue=w567, error in (no error)=w573) -> (error out=w565:errorcluster)  [unwired: 1 in, 2 out]
        n238 = Release Notifier(notifier=w566, error in (no error)=w565) -> (error out=w564:errorcluster)  [unwired: 1 in, 2 out]
        n239 = Release Queue(queue=w563, error in (no error)=w564) -> (error out=w559:errorcluster)  [unwired: 1 in, 2 out]
        n240 = call "Fire User Event - Stop.vi"("error in (no error)"=w559, "User Event - Stop"=w557) -> ("error out"=w558:errorcluster)  [unwired: 9 in]
      }
      frame "---Copy This Frame---" {
        # "Duplicate this frame when creating new messages.  Change this comment in the duplicated frame to describe this message."
        n241 = Merge Errors(w579) -> (w578:errorcluster)
      }
      frame "UpdateGraphSettings" {
        # "Duplicate this frame when creating new messages.  Change this comment in the duplicated frame to describe this message."
        n242 = Unbundle By Name(w580) -> ("Hardware Configuration.ActiveChannels"=w585:i32[], "Hardware Configuration.Display Rate"=w582:i32, "Hardware Configuration.ChannelNames"=w584:string[])
        n243 = Unbundle By Name(w580) -> ("Hardware Configuration"=→"Hardware Configuration":T1)
        n244 = Merge Errors(w623) -> (w594:errorcluster)
        n245 = for {
          tunnel: w585 -> [w634] mode=indexing
          tunnel: w584 -> [w629]
          tunnel: [w624] -> w583 mode=indexing
          n246 = Multiply(x=3, y=w634) -> (x*y=w633:i32)
          n247 = Index Array(array=w629, index=w633) -> (element=w628:string)
          n248 = String Length(string=w628) -> (length=w631:i32)
          n249 = Decrement(x=w631) -> (x-1=w630:i32)
          n250 = String Subset(string=w628, offset (0)=0, length (rest)=w630) -> (substring=w626:string)
          n251 = Bundle(waveform(sgl)[] [], "String"=w626, FALSE) -> (w624:cluster{waveform(sgl)[], "String":string, bool})  [unwired: 1 in]
        }
        n252 = Array Size(array=w585) -> (size(s)=w598:i32)
        n253 = property on="WD" class="Arr (strict)"(error in=w594, "Number of Rows"=w598) -> (error out=w605:errorcluster)  [unwired: 1 in, 1 out]
        n254 = property on="Pane" class="Pane"(error in=w605) -> (error out=w606:errorcluster, "ContentBnds"=w607:T9)  [unwired: 1 in, 1 out]
        n255 = Unbundle By Name(w607) -> ("Right"=w618:i16, "Bottom"=w620:i16, "Left"=w617:i16, "Top"=w619:i16)
        n256 = Subtract(x=w618, y=w617) -> (x-y=w616:i16)
        n257 = Subtract(x=w620, y=w619) -> (x-y=w615:i16)
        n258 = expression code="abs(x)-100"(w616) -> (w612:i16)
        n259 = Subtract(x=w615, y=w600) -> (x-y=w614:i16)
        n260 = Multiply(x=w598, y=3) -> (x*y=w602:i32)
        n261 = Divide(x=w614, y=w598) -> (x/y=w610:dbl)
        n262 = property on="Chart Length[s]" class="DigNum (strict)"() -> ("Value"=w586:dbl)  [unwired: 2 in, 2 out]
        n263 = To Long Integer(number=w610) -> (32bit integer=w609:i32)
        n264 = property on="Graph" class="WFGraph (strict)"() -> ("Plot Area Size"=w592:T14, "XScale.Range"=w591:T8)  [unwired: 2 in, 2 out]
        n265 = Subtract(x=w609, y=w599) -> (x-y=w608:i32)
        n266 = Multiply(x=w586, y=w582) -> (x*y=w604:dbl)
        n267 = Bundle By Name(cluster=w591, "Minimum"=0.0, "Maximum"=w586, "Increment"=1.0, "Minor Increment"=0.1) -> (w590:T8)
        n268 = Bundle(cluster=w592, "Width"=w612, "Height"=w608) -> (w613:T14)
        n269 = local write "WD"(w583) -> ()
        n270 = property on="Graph" class="WFGraph (strict)"(error in=w606, "Plot Area Size"=w613, "XScale.Range"=w590) -> (error out=w611:errorcluster)  [unwired: 1 in, 1 out]
        n271 = To Long Integer(number=w604) -> (32bit integer=w603:i32)
        n272 = invoke on="WD" class="Arr (strict)" method="FitControlToPane"(error in=w611) -> (error out=w596:errorcluster)  [unwired: 2 in, 2 out]
        n273 = Equal To 0?(x=w603) -> (x = 0?=w593:bool)
        n274 = Bundle(w603, w602) -> (w597:cluster{i32, i32})  [unwired: 1 in]
        n275 = case shown="False" w593 {
          tunnel: w597 -> [w637 _]
          tunnel: [w636 w643] -> w595
          tunnel: w596 -> [w641 w643]
          frame False {
            n276 = call-poly <userlib>:"Circular Buffer.vi"("Buffer Size"=T12 {"Samples per Channel"=0, "Channels"=0}, "error in (no error)"=w641, "Operation"=Circular_Buffer_Operations."Initialize") -> ("error out"=w640:errorcluster)  [unwired: 5 in, 3 out]
            n277 = call-poly <userlib>:"Circular Buffer.vi"("Buffer Size"=w637, "error in (no error)"=w640, "Operation"=Circular_Buffer_Operations."Initialize") -> ("error out"=w636:errorcluster)  [unwired: 5 in, 3 out]
          }
          frame True {
          }
        }
      }
      frame Default {
        # "'Default' case only runs if there is a message that isn't defined in any of the other cases.  Output a programming error."
        n278 = xnode "Error Ring"("parameter 0"=w645) -> ("error out"=w646:errorcluster)
      }
    }
    n279 = Unbundle By Name(w283) -> ("Hardware Configuration"=w282:T1)
    n280 = call "Error Handler - Message Handling Loop.vi"("error in (no error)"=w290, "Message Queue"=w281) -> ("dup error in"=w289:errorcluster)  [unwired: 8 in, 1 out]
    n281 = local write "Hardware Configuration"(w282) -> ()
  }
  n282 = Unregister For Events(event registration refnum=w19, error in=w27) -> (error out=w20:errorcluster)
  n283 = Merge Errors(w20, w28, w24, w21) -> (w26:errorcluster)
  n284 = property on="Hardware Configuration" class="Clust (strict)"("Visible"=FALSE) -> ()  [unwired: 2 in, 2 out]
  n285 = call "Destroy User Event - Stop.vi"("error in (no error)"=w26, "User Event - Stop"=w2) -> ("error out"=w12:errorcluster)  [unwired: 9 in]
  n286 = disable-structure shown="RUN_TIME_ENGINE==True" {
    disable-tunnel: w12 -> [_ _]
    frame condition #0 {
      # "Call Quit LabVIEW if running as a built application."
      n287 = Quit LabVIEW() -> ()  [unwired: 1 in]
    }
    frame condition #1 (active) {
    }
  }
